vi "Excel_Da.vi"(6 "(1_IL,0_uL)":bool, 7 "KG20":dbl[](array[numeric]), 8 "error in (no error)":errorcluster, 10 "Report path in":path, 11 "Test?":bool) -> (0 "error out":errorcluster, 2 "Report path out":path)   [LabVIEW 2015]
doc: "向报表的表格中输入IL（黑心圆）和uL（白底方）"
panel:
  in  "Start(-1,-1)":cluster{"row":i32, "column":i32}
  in  "excel application":refnum<k7>
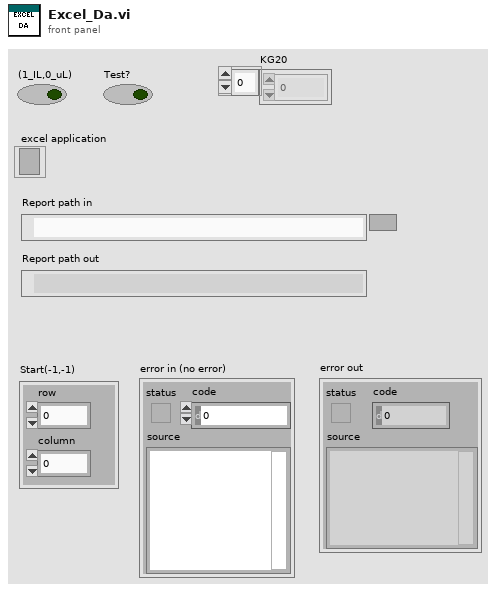
[diagram p1: front panel]
types:
  T1 = cluster{"Application":refnum<k7>, "Workbook":refnum<k7>, "Worksheet":refnum<k7>, "Shapes":refnum<k7>, "Worksheets":refnum<k7>}
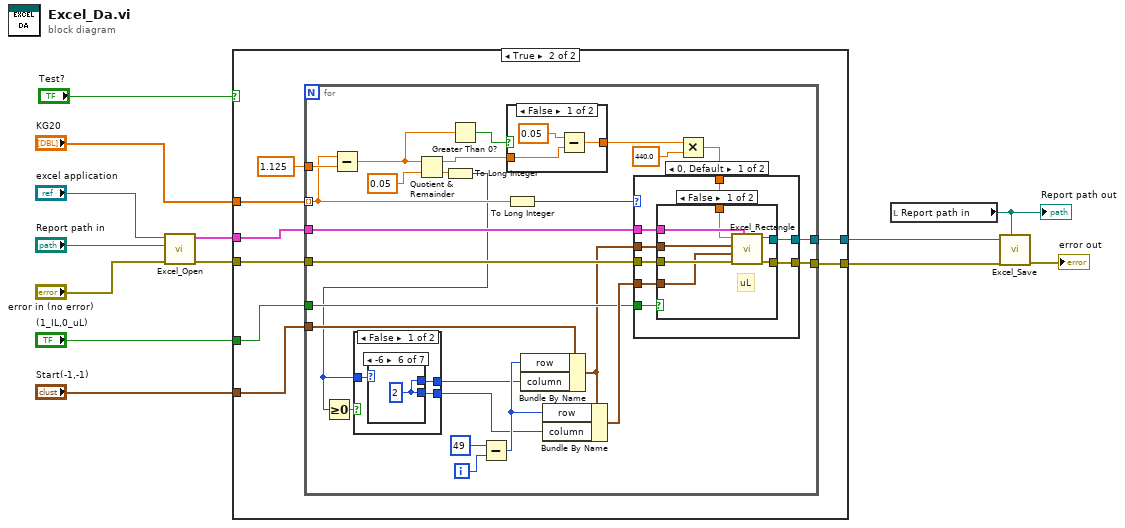
[diagram p0: block diagram]
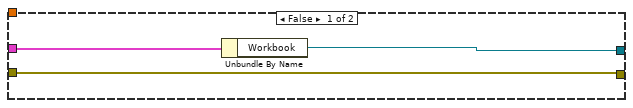
[diagram p2: hidden frame]
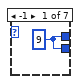
[diagram p3: hidden frame]
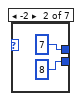
[diagram p4: hidden frame]
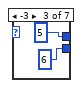
[diagram p5: hidden frame]
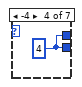
[diagram p6: hidden frame]
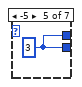
[diagram p7: hidden frame]
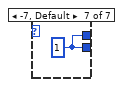
[diagram p8: hidden frame]
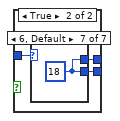
[diagram p9: hidden frame]
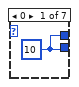
[diagram p10: hidden frame]
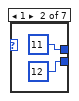
[diagram p11: hidden frame]
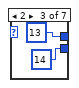
[diagram p12: hidden frame]
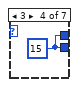
[diagram p13: hidden frame]
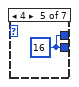
[diagram p14: hidden frame]
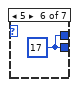
[diagram p15: hidden frame]
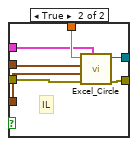
[diagram p16: hidden frame]
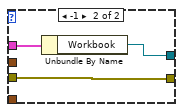
[diagram p17: hidden frame]
diagram:
  n1 = call "Excel_Open.vi"("error in (no error)"="error in (no error)", "template (empty)"="Report path in", "excel application"="excel application") -> ("error out"=w10:errorcluster, "references"=w11:T1)  [unwired: 7 in]
  n2 = case shown="True" "Test?" {
    tunnel: w11 -> [w15 w23]
    tunnel: w10 -> [w16 w22]
    tunnel: [w16 w21] -> w9
    tunnel: [w14 w20] -> w8
    tunnel: "KG20" -> [_ w19]
    tunnel: "(1_IL,0_uL)" -> [_ w18]
    tunnel: "Start(-1,-1)" -> [_ w17]
    frame False {
      n3 = Unbundle By Name(w15) -> ("Workbook"=w14:refnum<k7>)
    }
    frame True {
      n4 = for {
        tunnel: 1.125 ("DA") -> [w50]
        tunnel: w17 -> [w48]
        tunnel: w23 -> [w36]
        tunnel: w22 -> [w35]
        tunnel: [w34] -> w21
        tunnel: [w33] -> w20
        tunnel: w18 -> [w31]
        tunnel: w19 -> [w30] mode=indexing
        i -> [w46]
        n5 = Subtract(x=w30, y=w50) -> (x-y=w42:dbl)
        n6 = Quotient & Remainder(x=w42, y=0.05) -> (x-y*floor(x/y)=w40:dbl, floor(x/y)=w32:dbl)
        n7 = To Long Integer(number=w32) -> (32bit integer=w25:i32)
        n8 = Greater Or Equal To 0?(x=w25) -> (x >= 0?=w26:bool)
        n9 = case shown="False" w26 {
          tunnel: [w53 w65] -> w44
          tunnel: [w52 w64] -> w27
          tunnel: w25 -> [w51 w63]
          frame False {
            n10 = case shown="-6" w51 {
              tunnel: [w54 7 ("column") 5 ("column") w59 w60 w61 w62] -> w53
              tunnel: [w54 8 ("column") 6 ("column") w59 w60 w61 w62] -> w52
              frame -1 {
                w54 = 9 ("column")
              }
              frame -2 {
              }
              frame -3 {
              }
              frame -4 {
                w59 = 4 ("column")
              }
              frame -5 {
                w60 = 3 ("column")
              }
              frame -6 {
                w61 = 2 ("column")
              }
              frame -7, Default {
                w62 = 1 ("column")
              }
            }
          }
          frame True {
            n11 = case shown="6, Default" w63 {
              tunnel: [w66 11 ("column") 13 ("column") w71 w72 w73 w74] -> w65
              tunnel: [w66 12 ("column") 14 ("column") w71 w72 w73 w74] -> w64
              frame 0 {
                w66 = 10 ("row")
              }
              frame 1 {
              }
              frame 2 {
              }
              frame 3 {
                w71 = 15 ("column")
              }
              frame 4 {
                w72 = 16 ("column")
              }
              frame 5 {
                w73 = 17 ("column")
              }
              frame 6, Default {
                w74 = 18 ("column")
              }
            }
          }
        }
        n12 = Greater Than 0?(x=w42) -> (x > 0?=w41:bool)
        n13 = Subtract(x=49 ("column"), y=w46) -> (x-y=w45:i32)
        n14 = case shown="False" w41 {
          tunnel: w40 -> [w101 w103]
          tunnel: [w102 w103] -> w39
          frame False {
            n15 = Subtract(x=0.05 ("y"), y=w101) -> (x-y=w102:dbl)
          }
          frame True {
          }
        }
        n16 = To Long Integer(number=w30) -> (32bit integer=w29:i32)
        n17 = Bundle By Name(cluster=w48, "row"=w45, "column"=w44) -> (w28:cluster{"row":i32, "column":i32})
        n18 = Bundle By Name(cluster=w28, "row"=w45, "column"=w27) -> (w43:cluster{"row":i32, "column":i32})
        n19 = Multiply(x=w39, y=440.0) -> (x*y=w37:dbl)
        n20 = case shown="0, Default" w29 {
          tunnel: w43 -> [w75 _]
          tunnel: w28 -> [w76 _]
          tunnel: w37 -> [w82 _]
          tunnel: w36 -> [w81 w98]
          tunnel: w35 -> [w80 w99]
          tunnel: [w79 w99] -> w34
          tunnel: [w78 w97] -> w33
          tunnel: w31 -> [w77 _]
          frame 0, Default {
            n21 = case shown="False" w77 {
              tunnel: w75 -> [w83 w96]
              tunnel: w76 -> [w85 w95]
              tunnel: w82 -> [w86 w94]
              tunnel: w81 -> [w87 w93]
              tunnel: w80 -> [w84 w92]
              tunnel: [w88 w91] -> w79
              tunnel: [w89 w90] -> w78
              frame False {
                # "uL"
                n22 = call "Excel_Rectangle.vi"("references"=w87, "error in"=w84, "End(-1,-1)"=w83, "start(-1,-1)"=w85, "Left"=w86) -> ("error out"=w88:errorcluster, "Workbook"=w89:refnum<k7>)  [unwired: 5 in]
              }
              frame True {
                # "IL"
                n23 = call "Excel_Circle.vi"("references"=w93, "error in"=w92, "End(-1,-1)"=w96, "start(-1,-1)"=w95, "Left"=w94) -> ("error out"=w91:errorcluster, "Workbook"=w90:refnum<k7>)  [unwired: 5 in]
              }
            }
          }
          frame -1 {
            n24 = Unbundle By Name(w98) -> ("Workbook"=w97:refnum<k7>)
          }
        }
      }
    }
  }
  n25 = local read "Report path in"() -> (w2:path)
  "Report path out" <- w2
  n26 = call "Excel_Save.vi"("report file path"=w2, "error in (no error)"=w9, "Excel._Workbook"=w8) -> ("error out"=→"error out":errorcluster)  [unwired: 8 in]
